vi "Control - Generic - EGR Host.vi"() -> ()   [LabVIEW 2015, in "ECS-Host.lvlib"]
uses:
  ECS-Host.lvlib
  <vilib>/addons/Software Calibration Management/XControls/TBL2D.xctl
panel:
  out "HighPEGRPsn_PIDOut":sgl caption="[]"
  out "HighPEGRPsn_FF":sgl caption="[]"
  in  "HighPEGRPsn_FFMan":sgl caption="[]"
  out "HighPEGRPsn_Calc":sgl caption="[]"
  out "LowPEGRPsn_Des":sgl caption="[%Open]"
  out "LowPEGRPsn_TblOut":sgl caption="[]"
  in  "LowPEGRPsn_Tbl":cluster{"X":sgl[], "Y":sgl[], "Z":sgl[][]}(xcontrol) caption="[]"
  in  "HighPEGRPsn_FFManE":bool
  out "HighPEGRPsn_FFTblOut":sgl caption="[%Open]"
  in  "HighPEGRPsn_Man":sgl caption="[]"
  in  "HighPEGRPsn_ManE":bool
  in  "HighPEGRPsn_Max":sgl caption="[]"
  in  "HighPEGRPsn_Min":sgl caption="[]"
  in  "LowPEGRPsn_Min":sgl caption="[]"
  in  "LowPEGRPsn_Max":sgl caption="[]"
  in  "LowPEGRPsn_ManE":bool
  out "HighPEGRPsn_Des":sgl caption="[%Open]"
  in  "LowPEGRPsn_Man":sgl caption="[]"
  in  "HighPEGRPsn_PIDE":bool
  in  "HighPEGRPsn_Td":sgl caption="[min]"
  in  "HighPEGRPsn_Ti":sgl caption="[min]"
  in  "HighPEGRPsn_Kp":sgl caption="[%/mg/cyc]"
  in  "HighPEGRPsn_PIDMin":sgl caption="[%]"
  in  "HighPEGRPsn_PIDMax":sgl caption="[%]"
  out "EGRMass_Des":sgl caption="[mg/cyc]"
  in  "EGRMassStp_ManE":bool
  in  "EGRMassStp_Tbl":cluster{"X":sgl[], "Y":sgl[], "Z":sgl[][]}(xcontrol) caption="[kg/hr]"
  in  "HighPEGRPsn_FFTbl":cluster{"X":sgl[], "Y":sgl[], "Z":sgl[][]}(xcontrol) caption="[]"
  out "EGRMassStp_TblOut":sgl caption="[]"
  in  "EGRMassStp_Man":sgl caption="[]"
  # "EGR Setpoint"
  # "High Pressure EGR Position PID"
  # "High Pressure EGR Position"
  # "Low Pressure EGR Position"
  # "High Pressure EGR Position \nFeed Forward"
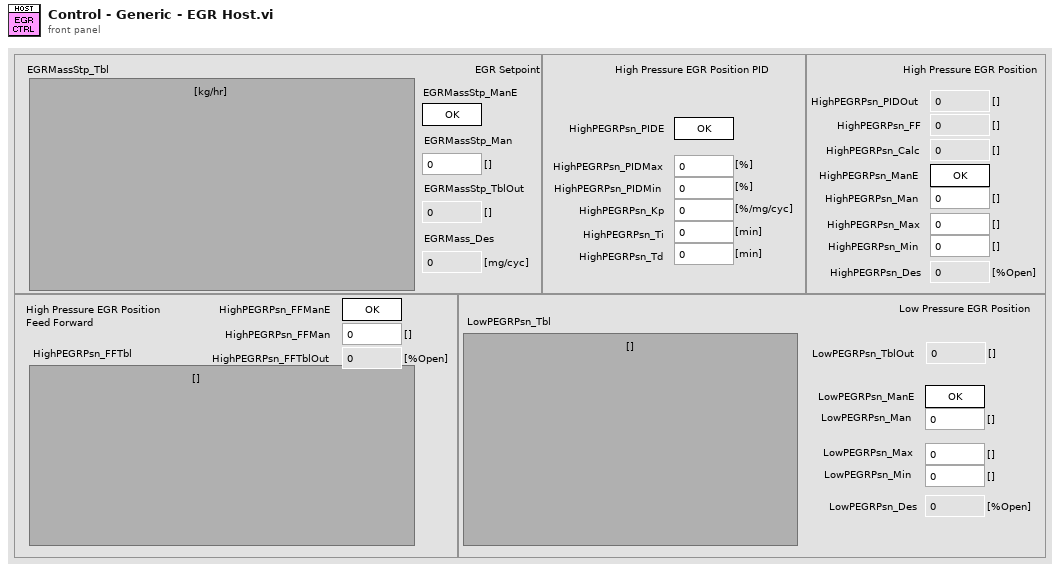
[diagram p1: front panel]
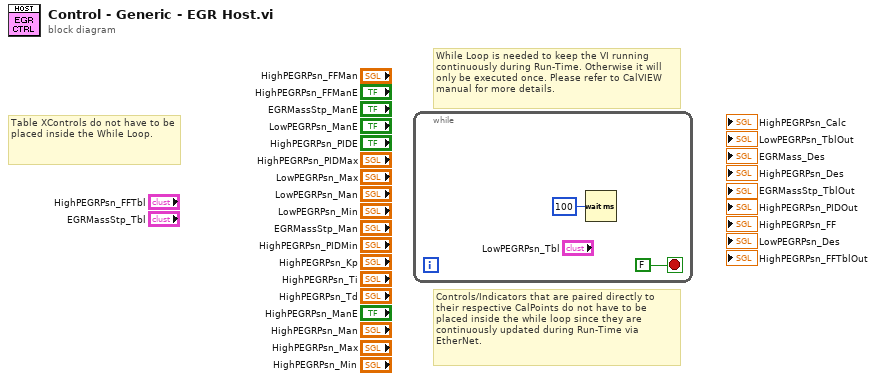
[diagram p0: block diagram]
diagram:
  # "Controls/Indicators that are paired directly to their respective CalPoints do not have to be placed inside the while loop since they are continuously updated during Run-Time via EtherNet."
  # "Table XControls do not have to be placed inside the While Loop."
  # "While Loop is needed to keep the VI running\ncontinuously during Run-Time. Otherwise it will only be executed once. Please refer to CalVIEW manual for more details."
  n1 = while {
    stop <- FALSE stop-if-true
    n2 = Wait (ms)(milliseconds to wait=u32 100) -> ()  [unwired: 1 out]
  }
